vi "Check Chassis Timing.vi"(8 "error in (no error)":errorcluster, 11 "Device Item Ref in":T1 format="%.0x") -> (0 "error out":errorcluster, 3 "Device Item Ref out":T1 format="%.0x")   [LabVIEW 2010, in "PXIe-433x Custom Device.lvlib"]
uses:
  PXIe-433x Custom Device.lvlib
  <vilib>/NI Veristand/Custom Device API/Custom Device Item Ref.ctl
  NationalInstruments.VeriStand.SystemStorage
  Global.vi
  <vilib>/NI Veristand/Custom Device API/Set Item Property (Boolean).vi
  <vilib>/NI Veristand/Custom Device API/Set Item Property (U32).vi
  <vilib>/NI Veristand/Custom Device API/Custom Device API.lvlib
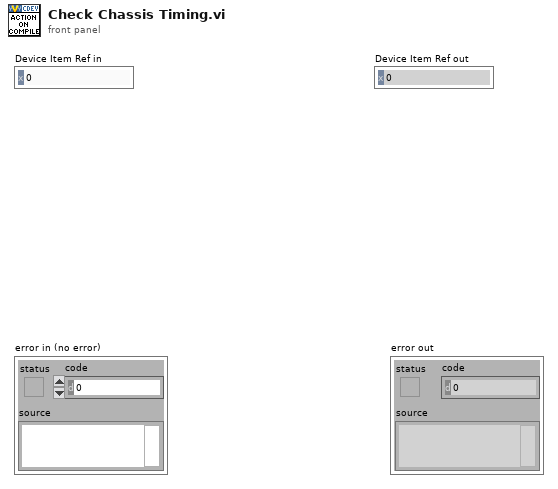
[diagram p1: front panel]
types:
  T1 = typedef "Custom Device API.lvlib/Custom Device Item Ref.ctl" = u64
  T2 = typedef "Custom Device API.lvlib/Custom Device Pointer.ctl" = refnum<k24>
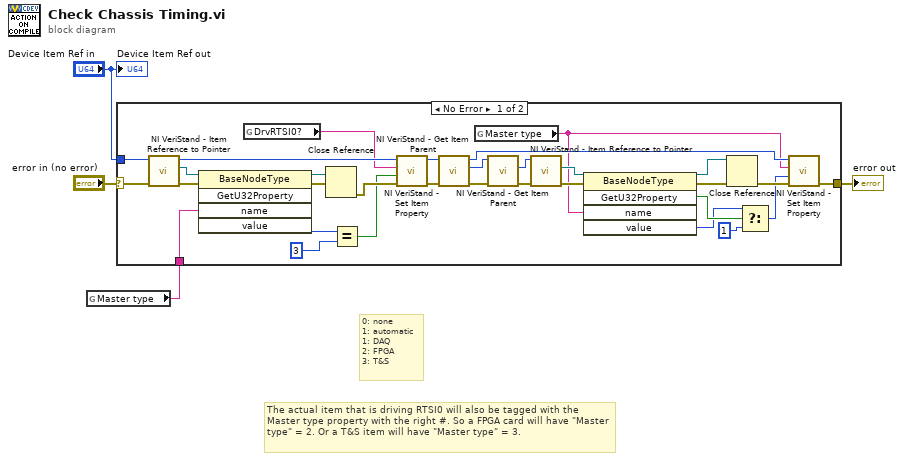
[diagram p0: block diagram]
diagram:
  # "The actual item that is driving RTSI0 will also be tagged with the Master type property with the right #. So a FPGA card will have \"Master type\" = 2. Or a T&S item will have \"Master type\" = 3."
  # "0: none\n1: automatic\n1: DAQ\n2: FPGA\n3: T&S"
  n1 = global read "Global.vi" "Master type"() -> (w1:string)
  n2 = case shown="No Error" "error in (no error)" {
    selector: "error in (no error)" -> [w19 w36]
    tunnel: [w24 w36] -> w3
    tunnel: "Device Item Ref in" -> [w18 _]
    tunnel: w1 -> [w15 _]
    frame No Error {
      n3 = call <vilib>:"NI VeriStand - Item Reference to Pointer.vi"("error in (no error)"=w19, "Item Ref in"=w18) -> ("error out"=w16:errorcluster, "Node Pointer"=w17:T2, "Item Ref out"=w12:T1)  [unwired: 6 in, 1 out]
      n4 = invoke class="BaseNodeType" method="GetU32Property"(reference=w17, error in=w16, "name"=w15) -> (reference out=w13:T2, error out=w14:errorcluster, "value"=w9:u32)  [unwired: 2 in, 2 out]
      n5 = global read "Global.vi" "DrvRTSI0?"() -> (w10:string)
      n6 = Close Reference(reference=w13, error in (no error)=w14) -> (error out=w11:errorcluster)
      n7 = Equal?(x=w9, y=u32 3) -> (x = y?=w7:bool)
      n8 = call-poly <vilib>:"NI VeriStand - Set Item Property.vi"("error in (no error)"=w11, "Value"=w7, "Property Name"=w10, "Item Ref in"=w12) -> ("error out"=w6:errorcluster, "Item Ref out"=w5:T1)  [unwired: 5 in, 1 out]
      n9 = call <vilib>:"NI VeriStand - Get Item Parent.vi"("error in (no error)"=w6, "Item Ref in"=w5) -> ("error out"=w35:errorcluster, "Parent Ref"=w34:T1, "Item Ref out"=w26:T1)  [unwired: 6 in, 1 out]
      n10 = global read "Global.vi" "Master type"() -> (w25:string)
      n11 = call <vilib>:"NI VeriStand - Get Item Parent.vi"("error in (no error)"=w35, "Item Ref in"=w34) -> ("error out"=w33:errorcluster, "Parent Ref"=w32:T1)  [unwired: 6 in, 2 out]
      n12 = call <vilib>:"NI VeriStand - Item Reference to Pointer.vi"("error in (no error)"=w33, "Item Ref in"=w32) -> ("error out"=w31:errorcluster, "Node Pointer"=w30:T2)  [unwired: 6 in, 2 out]
      n13 = invoke class="BaseNodeType" method="GetU32Property"(reference=w30, error in=w31, "name"=w25) -> (reference out=w28:T2, error out=w29:errorcluster, "GetU32Property"=w23:bool, "value"=w22:u32)  [unwired: 2 in, 1 out]
      n14 = Close Reference(reference=w28, error in (no error)=w29) -> (error out=w27:errorcluster)
      n15 = Select(t=w22, s=w23, f=u32 1) -> (s? t:f=w21:u32)
      n16 = call-poly <vilib>:"NI VeriStand - Set Item Property.vi"("error in (no error)"=w27, "Value"=w21, "Property Name"=w25, "Item Ref in"=w26) -> ("error out"=w24:errorcluster)  [unwired: 5 in, 2 out]
    }
    frame Error {
    }
  }
  "error out" <- w3
  "Device Item Ref out" <- "Device Item Ref in"
